vi "AddStep.vi"(8 "error in (no error)":errorcluster, 9 "StepName":string, 10 "StepType":T1, 11 "Project.lvclass In":refnum<class "Project.lvclass">) -> (0 "error out":errorcluster, 3 "Project.lvclass Out":refnum<class "Project.lvclass">)   [LabVIEW 2014, in "Project.lvclass"]
uses:
  Project.lvclass
  StepData/Control/StepTypeEnum.ctl
  StepSetupDataTypeDefine.ctl
  StepData/Control/AllStepTypeData.ctl
  StepData/Control/MoveData.ctl
  StepData/Control/MeasureData.ctl
  Project.lvclass/Project.ctl
  StepData/StepData.lvclass
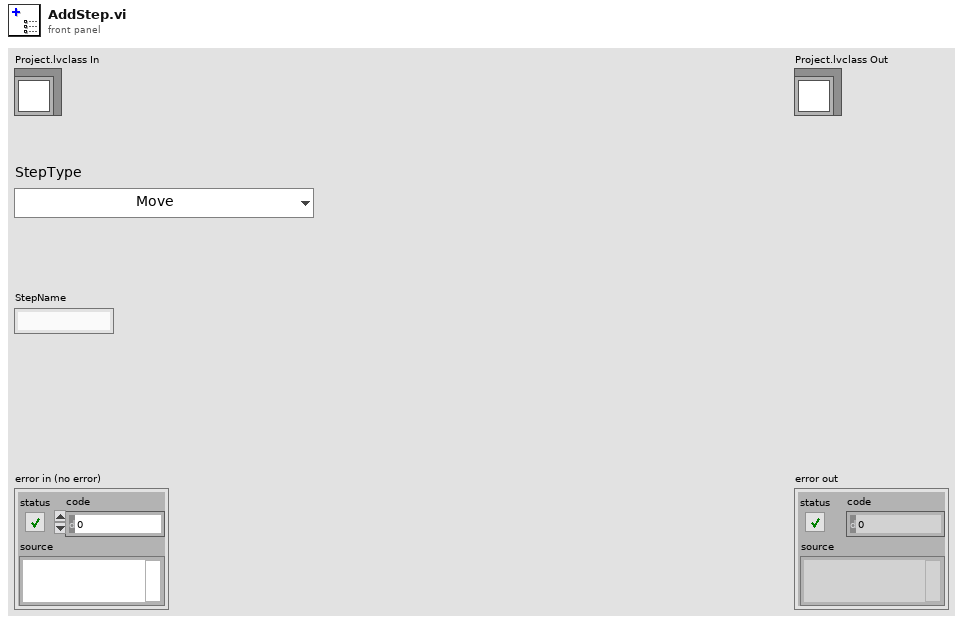
[diagram p1: front panel]
types:
  T1 = typedef "StepData.lvclass/StepTypeEnum.ctl" = enum16{"Move", "Measure"}
  T2 = typedef "Project.lvclass/StepSetupDataTypeDefine.ctl" = cluster{"AllStepTypeData":T3}[]
  T3 = typedef "StepData.lvclass/AllStepTypeData.ctl" = cluster{"StepName":string, "StepTypeEnum":T1, "MoveData":T4, "MeasureData":T5}
  T4 = typedef "StepData.lvclass/MoveData.ctl" = cluster{"Axis":u16, "Position":dbl, "Speed":dbl, "Acc/Dec":dbl, "Mode":u16}
  T5 = typedef "StepData.lvclass/MeasureData.ctl" = cluster{"Sensor No.":i32, "Log?":bool}
  T6 = typedef "Project.lvclass/ProjectDataTableTypeDefine.ctl" = string[][]
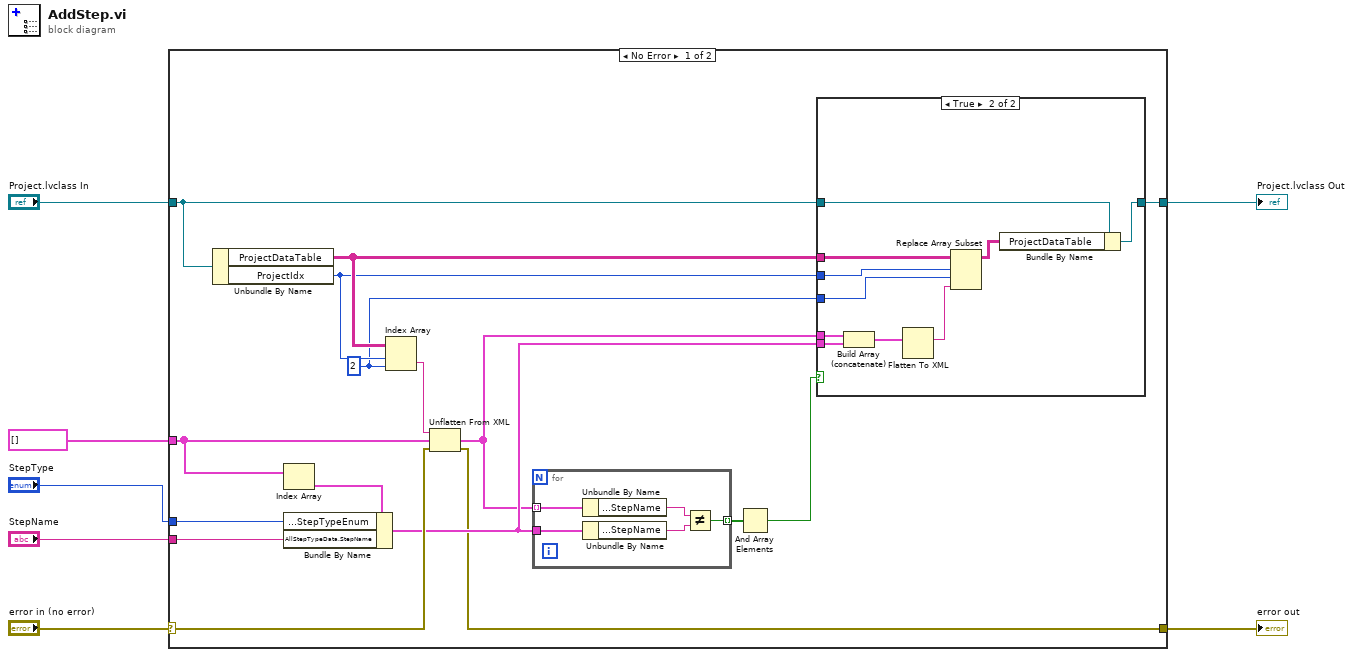
[diagram p0: block diagram]
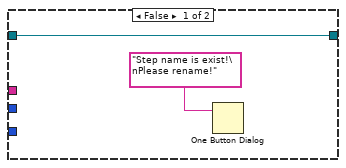
[diagram p2: hidden frame]
diagram:
  n1 = case shown="No Error" "error in (no error)" {
    selector: "error in (no error)" -> [w15 w42]
    tunnel: [w9 w42] -> w6
    tunnel: "Project.lvclass In" -> [w20 w41]
    tunnel: "StepName" -> [w17 _]
    tunnel: [w19 w41] -> w3
    tunnel: T2 [] ("StepSetupClusterArray") -> [w12 _]
    tunnel: "StepType" -> [w14 _]
    frame No Error {
      w21 = 2 ("disabled index (col)")
      n2 = Unbundle By Name(w20) -> ("ProjectDataTable"=w23:T6, "ProjectIdx"=w22:i32)
      n3 = Index Array(array=w12) -> (element=w18:cluster{"AllStepTypeData":T3})  [unwired: 1 in]
      n4 = Bundle By Name(cluster=w18, "AllStepTypeData.StepTypeEnum"=w14, "AllStepTypeData.StepName"=w17) -> (w11:cluster{"AllStepTypeData":T3})
      n5 = Index Array(array=w23, index (row)=w22, index (col)=w21) -> (element=w16:string)
      n6 = Unflatten From XML(xml string=w16, type=w12, error in (no error)=w15) -> (value=w8:T2, error out=w9:errorcluster)
      n7 = for {
        tunnel: w8 -> [w28] mode=indexing
        tunnel: w11 -> [w27]
        tunnel: [w24] -> w13 mode=indexing
        n8 = Unbundle By Name(w28) -> ("AllStepTypeData.StepName"=w26:string)
        n9 = Unbundle By Name(w27) -> ("AllStepTypeData.StepName"=w25:string)
        n10 = Not Equal?(x=w26, y=w25) -> (x != y?=w24:bool)
      }
      n11 = And Array Elements(Boolean array=w13) -> (logical AND=w10:bool)
      n12 = case shown="True" w10 {
        tunnel: w23 -> [_ w40]
        tunnel: w22 -> [_ w39]
        tunnel: w21 -> [_ w38]
        tunnel: w20 -> [w30 w37]
        tunnel: [w30 w35] -> w19
        tunnel: w8 -> [_ w33]
        tunnel: w11 -> [_ w32]
        frame False {
          n13 = One Button Dialog(message="Step name is exist!\nPlease rename!") -> ()  [unwired: 1 in, 1 out]
        }
        frame True {
          n14 = Build Array (concatenate)(w33, w32) -> (w34:T2)
          n15 = Flatten To XML(anything=w34) -> (xml string=w31:string)
          n16 = Replace Array Subset(array=w40, new element=w31, index (row)=w39, index (col)=w38) -> (w36:T6)
          n17 = Bundle By Name(cluster=w37, "ProjectDataTable"=w36) -> (w35:refnum<class "Project.lvclass">)
        }
      }
    }
    frame Error {
    }
  }
  "error out" <- w6
  "Project.lvclass Out" <- w3
